vi "Configuration Editor.vi"() -> ()   [LabVIEW 2013]
doc: "This VI allows the user to create or edit an existing file located in the same directory as the the CAT Panel or the CAT Configuration Editor. It begins by opening the encrypted configuration file cat panel.cfg. The file is decrypted and then decrypted text is written to a temporary file located in the directory C:\\temp (the temporary file is called cat panel.tmp and is deleted upon successful edit of the configuration file). If the configuration file exists, then data is read into the front panel controls. When the user edits and saves the data on the front panel, the data is queued up for writing in the configuration files. Upon exit, the saved configuration data is read, the temporary file is deleted, the saved data is encrypted and written to the file cat pane.cfg."
uses:
  Type Defs/AD Settings.ctl
  Type Defs/Output Values.ctl
  Type Defs/Output Switches.ctl
  Type Defs/CO2 Settings.ctl
  Type Defs/Named Final Output name list ordered.ctl
  <vilib>/Utility/config.llb/Read Key (I32).vi
  <vilib>/Utility/config.llb/Read Key (Double).vi
  <vilib>/Utility/config.llb/Read Key (Boolean).vi
  <vilib>/Utility/config.llb/Read Key (String).vi
  <vilib>/Utility/config.llb/Write Key (I32).vi
  <vilib>/Utility/config.llb/Write Key (Double).vi
  <vilib>/Utility/config.llb/Write Key (Boolean).vi
  <vilib>/Utility/config.llb/Write Key (String).vi
  <vilib>/Utility/config.llb/NI_LVConfig.lvlib
panel:
  out "Saved?":bool
  in  "close":bool
  in  "Save":bool
  in  "tab":T1(tab)=enum."Hypoxic AD Settings"
  in  "Hyperoxic AD Settings":T2={"Set Point Force"={"A-1,  1"=inf, "A-3,  2"=inf, "A-4, 3"=inf, "A-5, 4"=5790.0, "ABCD-7, 5"=inf, "A-8, 6"=inf, "B-1,  7"=5790.0, "B-3, 8"=5790.0, "B-4,  9"=inf, "B-5, 10"=5790.0, "B-8, 11"=inf, "C-1, 12"=inf, "C-3, 13"=inf, "C-4, 14"=inf, "C-5,  15"=5790.0, "C-8, 16"=inf, "D-1, 17"=inf, "D-3, 18"=inf, "D-4,  19"=inf, "D-5,  20"=inf, "D-8,  21"=inf}, "Run A1"={"A-1,  1"=inf, "A-3,  2"=inf, "A-4, 3"=3.0, "A-5, 4"=inf, "ABCD-7, 5"=67.0, "A-8, 6"=630.0, "B-1,  7"=-30.0, "B-3, 8"=-30.0, "B-4,  9"=3.0, "B-5, 10"=inf, "B-8, 11"=630.0, "C-1, 12"=-60.0, "C-3, 13"=-60.0, "C-4, 14"=3.0, "C-5,  15"=inf, "C-8, 16"=630.0, "D-1, 17"=inf, "D-3, 18"=-30.0, "D-4,  19"=-60.0, "D-5,  20"=630.0, "D-8,  21"=930.0}, "Run A2"={"A-1,  1"=inf, "A-3,  2"=inf, "A-4, 3"=-3.0, "A-5, 4"=inf, "ABCD-7, 5"=60.0, "A-8, 6"=610.0, "B-1,  7"=-100.0, "B-3, 8"=-100.0, "B-4,  9"=-3.0, "B-5, 10"=inf, "B-8, 11"=610.0, "C-1, 12"=-120.0, "C-3, 13"=-120.0, "C-4, 14"=-3.0, "C-5,  15"=inf, "C-8, 16"=610.0, "D-1, 17"=inf, "D-3, 18"=-100.0, "D-4,  19"=-120.0, "D-5,  20"=610.0, "D-8,  21"=910.0}, "Hold A3"={"A-1,  1"=0.0, "A-3,  2"=0.0, "A-4, 3"=3.0, "A-5, 4"=inf, "ABCD-7, 5"=67.0, "A-8, 6"=630.0, "B-1,  7"=-150.0, "B-3, 8"=-150.0, "B-4,  9"=3.0, "B-5, 10"=inf, "B-8, 11"=630.0, "C-1, 12"=-300.0, "C-3, 13"=-300.0, "C-4, 14"=3.0, "C-5,  15"=inf, "C-8, 16"=630.0, "D-1, 17"=0.0, "D-3, 18"=-150.0, "D-4,  19"=-300.0, "D-5,  20"=630.0, "D-8,  21"=930.0}, "Hold A4"={"A-1,  1"=-150.0, "A-3,  2"=-150.0, "A-4, 3"=-3.0, "A-5, 4"=inf, "ABCD-7, 5"=60.0, "A-8, 6"=610.0, "B-1,  7"=-250.0, "B-3, 8"=-250.0, "B-4,  9"=-3.0, "B-5, 10"=inf, "B-8, 11"=610.0, "C-1, 12"=-500.0, "C-3, 13"=-500.0, "C-4, 14"=-3.0, "C-5,  15"=inf, "C-8, 16"=610.0, "D-1, 17"=-150.0, "D-3, 18"=-250.0, "D-4,  19"=-500.0, "D-5,  20"=610.0, "D-8,  21"=910.0}, "High AD Diff "={"A-1, 1"=FALSE, "A-3, 2"=FALSE, "A-4, 3"=FALSE, "A-5, 4"=TRUE, "ABCD-7, 5"=FALSE, "A-8, 6"=TRUE, "B-1,  7"=FALSE, "B-3, 8"=FALSE, "B-4, 9"=FALSE, "B-5, 10"=TRUE, "B-8,  11"=TRUE, "C-1, 12"=FALSE, "C-3, 13"=FALSE, "C-4,  14"=FALSE, "C-5,  15"=TRUE, "C-8, 16"=TRUE, "D-1, 17"=FALSE, "D-3, 18"=FALSE, "D-4, 19"=FALSE, "D-5,  20"=TRUE, "D-8,  21"=TRUE}, "Delay S"={"A-1,  1"=30.0, "A-3,  2"=30.0, "A-4, 3"=1.0, "A-5, 4"=1.0, "ABCD-7, 5"=1.0, "A-8, 6"=1.0, "B-1,  7"=30.0, "B-3, 8"=30.0, "B-4,  9"=1.0, "B-5, 10"=1.0, "B-8, 11"=1.0, "C-1, 12"=30.0, "C-3, 13"=30.0, "C-4, 14"=1.0, "C-5,  15"=1.0, "C-8, 16"=1.0, "D-1, 17"=30.0, "D-3, 18"=30.0, "D-4,  19"=30.0, "D-5,  20"=1.0, "D-8,  21"=1.0}}
  in  "Hyperoxic CO2 Settings":T5={"Run C1"={"A-1,  1"=inf, "A-3,  2"=inf, "A-4, 3"=9600.0, "A-5, 4"=8800.0, "ABCD-7, 5"=9800.0, "A-8, 6"=9800.0, "B-1,  7"=3400.0, "B-3, 8"=3400.0, "B-4,  9"=9600.0, "B-5, 10"=8800.0, "B-8, 11"=9800.0, "C-1, 12"=1800.0, "C-3, 13"=1800.0, "C-4, 14"=9600.0, "C-5,  15"=8800.0, "C-8, 16"=9800.0, "D-1, 17"=inf, "D-3, 18"=3400.0, "D-4,  19"=1800.0, "D-5,  20"=9800.0, "D-8,  21"=9800.0}, "Run C2"={"A-1,  1"=inf, "A-3,  2"=inf, "A-4, 3"=9500.0, "A-5, 4"=8600.0, "ABCD-7, 5"=9700.0, "A-8, 6"=9700.0, "B-1,  7"=3000.0, "B-3, 8"=3000.0, "B-4,  9"=9500.0, "B-5, 10"=8600.0, "B-8, 11"=9700.0, "C-1, 12"=1400.0, "C-3, 13"=1400.0, "C-4, 14"=9500.0, "C-5,  15"=8600.0, "C-8, 16"=9700.0, "D-1, 17"=inf, "D-3, 18"=3000.0, "D-4,  19"=1400.0, "D-5,  20"=9700.0, "D-8,  21"=9700.0}, "Hold C3"={"A-1,  1"=1800.0, "A-3,  2"=1800.0, "A-4, 3"=9000.0, "A-5, 4"=8800.0, "ABCD-7, 5"=9800.0, "A-8, 6"=9800.0, "B-1,  7"=3400.0, "B-3, 8"=3400.0, "B-4,  9"=9000.0, "B-5, 10"=8800.0, "B-8, 11"=9800.0, "C-1, 12"=1800.0, "C-3, 13"=1800.0, "C-4, 14"=9000.0, "C-5,  15"=8800.0, "C-8, 16"=9800.0, "D-1, 17"=1800.0, "D-3, 18"=3400.0, "D-4,  19"=1800.0, "D-5,  20"=9800.0, "D-8,  21"=9800.0}, "Hold C4"={"A-1,  1"=1400.0, "A-3,  2"=1400.0, "A-4, 3"=8800.0, "A-5, 4"=8600.0, "ABCD-7, 5"=9700.0, "A-8, 6"=9700.0, "B-1,  7"=3000.0, "B-3, 8"=3000.0, "B-4,  9"=8800.0, "B-5, 10"=8600.0, "B-8, 11"=9700.0, "C-1, 12"=1400.0, "C-3, 13"=1400.0, "C-4, 14"=8800.0, "C-5,  15"=8600.0, "C-8, 16"=9700.0, "D-1, 17"=1400.0, "D-3, 18"=3000.0, "D-4,  19"=1400.0, "D-5,  20"=9700.0, "D-8,  21"=9700.0}, "High CO2 Forces"={"A-1, 1"=TRUE, "A-3, 2"=TRUE, "A-4, 3"=FALSE, "A-5, 4"=TRUE, "ABCD-7, 5"=FALSE, "A-8, 6"=TRUE, "B-1,  7"=TRUE, "B-3, 8"=TRUE, "B-4, 9"=FALSE, "B-5, 10"=TRUE, "B-8,  11"=TRUE, "C-1, 12"=TRUE, "C-3, 13"=TRUE, "C-4,  14"=FALSE, "C-5,  15"=TRUE, "C-8, 16"=TRUE, "D-1, 17"=TRUE, "D-3, 18"=TRUE, "D-4, 19"=TRUE, "D-5,  20"=TRUE, "D-8,  21"=TRUE}}
  in  "AD Settings":T2={"Set Point Force"={"A-1,  1"=inf, "A-3,  2"=inf, "A-4, 3"=inf, "A-5, 4"=5790.0, "ABCD-7, 5"=inf, "A-8, 6"=inf, "B-1,  7"=5790.0, "B-3, 8"=5790.0, "B-4,  9"=inf, "B-5, 10"=5790.0, "B-8, 11"=inf, "C-1, 12"=inf, "C-3, 13"=inf, "C-4, 14"=inf, "C-5,  15"=5790.0, "C-8, 16"=inf, "D-1, 17"=inf, "D-3, 18"=inf, "D-4,  19"=inf, "D-5,  20"=inf, "D-8,  21"=inf}, "Run A1"={"A-1,  1"=inf, "A-3,  2"=inf, "A-4, 3"=3.0, "A-5, 4"=inf, "ABCD-7, 5"=67.0, "A-8, 6"=630.0, "B-1,  7"=-30.0, "B-3, 8"=-30.0, "B-4,  9"=3.0, "B-5, 10"=inf, "B-8, 11"=630.0, "C-1, 12"=-60.0, "C-3, 13"=-60.0, "C-4, 14"=3.0, "C-5,  15"=inf, "C-8, 16"=630.0, "D-1, 17"=inf, "D-3, 18"=-30.0, "D-4,  19"=-60.0, "D-5,  20"=630.0, "D-8,  21"=930.0}, "Run A2"={"A-1,  1"=inf, "A-3,  2"=inf, "A-4, 3"=-3.0, "A-5, 4"=inf, "ABCD-7, 5"=60.0, "A-8, 6"=610.0, "B-1,  7"=-100.0, "B-3, 8"=-100.0, "B-4,  9"=-3.0, "B-5, 10"=inf, "B-8, 11"=610.0, "C-1, 12"=-120.0, "C-3, 13"=-120.0, "C-4, 14"=-3.0, "C-5,  15"=inf, "C-8, 16"=610.0, "D-1, 17"=inf, "D-3, 18"=-100.0, "D-4,  19"=-120.0, "D-5,  20"=610.0, "D-8,  21"=910.0}, "Hold A3"={"A-1,  1"=0.0, "A-3,  2"=0.0, "A-4, 3"=3.0, "A-5, 4"=inf, "ABCD-7, 5"=67.0, "A-8, 6"=630.0, "B-1,  7"=-150.0, "B-3, 8"=-150.0, "B-4,  9"=3.0, "B-5, 10"=inf, "B-8, 11"=630.0, "C-1, 12"=-300.0, "C-3, 13"=-300.0, "C-4, 14"=3.0, "C-5,  15"=inf, "C-8, 16"=630.0, "D-1, 17"=0.0, "D-3, 18"=-150.0, "D-4,  19"=-300.0, "D-5,  20"=630.0, "D-8,  21"=930.0}, "Hold A4"={"A-1,  1"=-150.0, "A-3,  2"=-150.0, "A-4, 3"=-3.0, "A-5, 4"=inf, "ABCD-7, 5"=60.0, "A-8, 6"=610.0, "B-1,  7"=-250.0, "B-3, 8"=-250.0, "B-4,  9"=-3.0, "B-5, 10"=inf, "B-8, 11"=610.0, "C-1, 12"=-500.0, "C-3, 13"=-500.0, "C-4, 14"=-3.0, "C-5,  15"=inf, "C-8, 16"=610.0, "D-1, 17"=-150.0, "D-3, 18"=-250.0, "D-4,  19"=-500.0, "D-5,  20"=610.0, "D-8,  21"=910.0}, "High AD Diff "={"A-1, 1"=FALSE, "A-3, 2"=FALSE, "A-4, 3"=FALSE, "A-5, 4"=TRUE, "ABCD-7, 5"=FALSE, "A-8, 6"=TRUE, "B-1,  7"=FALSE, "B-3, 8"=FALSE, "B-4, 9"=FALSE, "B-5, 10"=TRUE, "B-8,  11"=TRUE, "C-1, 12"=FALSE, "C-3, 13"=FALSE, "C-4,  14"=FALSE, "C-5,  15"=TRUE, "C-8, 16"=TRUE, "D-1, 17"=FALSE, "D-3, 18"=FALSE, "D-4, 19"=FALSE, "D-5,  20"=TRUE, "D-8,  21"=TRUE}, "Delay S"={"A-1,  1"=30.0, "A-3,  2"=30.0, "A-4, 3"=1.0, "A-5, 4"=1.0, "ABCD-7, 5"=1.0, "A-8, 6"=1.0, "B-1,  7"=30.0, "B-3, 8"=30.0, "B-4,  9"=1.0, "B-5, 10"=1.0, "B-8, 11"=1.0, "C-1, 12"=30.0, "C-3, 13"=30.0, "C-4, 14"=1.0, "C-5,  15"=1.0, "C-8, 16"=1.0, "D-1, 17"=30.0, "D-3, 18"=30.0, "D-4,  19"=30.0, "D-5,  20"=1.0, "D-8,  21"=1.0}}
  in  "CO2 Settings":T5={"Run C1"={"A-1,  1"=inf, "A-3,  2"=inf, "A-4, 3"=9600.0, "A-5, 4"=8800.0, "ABCD-7, 5"=9800.0, "A-8, 6"=9800.0, "B-1,  7"=3400.0, "B-3, 8"=3400.0, "B-4,  9"=9600.0, "B-5, 10"=8800.0, "B-8, 11"=9800.0, "C-1, 12"=1800.0, "C-3, 13"=1800.0, "C-4, 14"=9600.0, "C-5,  15"=8800.0, "C-8, 16"=9800.0, "D-1, 17"=inf, "D-3, 18"=3400.0, "D-4,  19"=1800.0, "D-5,  20"=9800.0, "D-8,  21"=9800.0}, "Run C2"={"A-1,  1"=inf, "A-3,  2"=inf, "A-4, 3"=9500.0, "A-5, 4"=8600.0, "ABCD-7, 5"=9700.0, "A-8, 6"=9700.0, "B-1,  7"=3000.0, "B-3, 8"=3000.0, "B-4,  9"=9500.0, "B-5, 10"=8600.0, "B-8, 11"=9700.0, "C-1, 12"=1400.0, "C-3, 13"=1400.0, "C-4, 14"=9500.0, "C-5,  15"=8600.0, "C-8, 16"=9700.0, "D-1, 17"=inf, "D-3, 18"=3000.0, "D-4,  19"=1400.0, "D-5,  20"=9700.0, "D-8,  21"=9700.0}, "Hold C3"={"A-1,  1"=1800.0, "A-3,  2"=1800.0, "A-4, 3"=9000.0, "A-5, 4"=8800.0, "ABCD-7, 5"=9800.0, "A-8, 6"=9800.0, "B-1,  7"=3400.0, "B-3, 8"=3400.0, "B-4,  9"=9000.0, "B-5, 10"=8800.0, "B-8, 11"=9800.0, "C-1, 12"=1800.0, "C-3, 13"=1800.0, "C-4, 14"=9000.0, "C-5,  15"=8800.0, "C-8, 16"=9800.0, "D-1, 17"=1800.0, "D-3, 18"=3400.0, "D-4,  19"=1800.0, "D-5,  20"=9800.0, "D-8,  21"=9800.0}, "Hold C4"={"A-1,  1"=1400.0, "A-3,  2"=1400.0, "A-4, 3"=8800.0, "A-5, 4"=8600.0, "ABCD-7, 5"=9700.0, "A-8, 6"=9700.0, "B-1,  7"=3000.0, "B-3, 8"=3000.0, "B-4,  9"=8800.0, "B-5, 10"=8600.0, "B-8, 11"=9700.0, "C-1, 12"=1400.0, "C-3, 13"=1400.0, "C-4, 14"=8800.0, "C-5,  15"=8600.0, "C-8, 16"=9700.0, "D-1, 17"=1400.0, "D-3, 18"=3000.0, "D-4,  19"=1400.0, "D-5,  20"=9700.0, "D-8,  21"=9700.0}, "High CO2 Forces"={"A-1, 1"=TRUE, "A-3, 2"=TRUE, "A-4, 3"=FALSE, "A-5, 4"=TRUE, "ABCD-7, 5"=FALSE, "A-8, 6"=TRUE, "B-1,  7"=TRUE, "B-3, 8"=TRUE, "B-4, 9"=FALSE, "B-5, 10"=TRUE, "B-8,  11"=TRUE, "C-1, 12"=TRUE, "C-3, 13"=TRUE, "C-4,  14"=FALSE, "C-5,  15"=TRUE, "C-8, 16"=TRUE, "D-1, 17"=TRUE, "D-3, 18"=TRUE, "D-4, 19"=TRUE, "D-5,  20"=TRUE, "D-8,  21"=TRUE}}
  in  "Buffer":sgl=1.0 min=0 max=100
  in  "Time Offset":dbl
  out "MD5 Hash":string
  in  "Setup Menu Passwords":T6
  out "Hash 3":string
  out "Hash 2":string
  out "Hash 1":string
  in  "Lockout Date 3":timestamp format="%<%H:%M\n%x>T"
  in  "Lockout Date 2":timestamp format="%<%H:%M\n%x>T"
  in  "Lockout Date 1":timestamp format="%<%H:%M\n%x>T"
  in  "custMaxAlt":dbl caption="Customer\nMax Altitude"
  in  "Alarm Setpoints":T7={"CalLimit"=10000.0, "SenseLimit"=10000.0, "CO2Lim"=10000.0, "AltLim"=10000.0, "Low O2 "=10000.0, "High O2 offset"=10000.0}
  in  "ID":string
  in  "Setpoint":sgl=10000.0
  in  "Mode":enum8{"Off", "Stby", "Hold", "Run"}(ring)=enum."Stby"
  in  "AltCalc":bool caption="Altitude Calculation"
  in  "Channel Names":T8={"A-1, 1"="Main", "A-3, 2"="Main", "A-4, 3"="Recirculation", "A-5, 4"="Scrubber", "A-7, 5"="Oxygen", "A-8, 6"="Vent", "B-1,  7"="Boost A", "B-3, 8"="Boost A", "B-4, 9"="Recirculation", "B-5, 10"="Scrubber", "B-8, 11"="Vent", "C-1, 12"="Boost B", "C-3, 13"="Boost B", "C-4, 14"="Recirculation", "C-5,  15"="Scrubber", "C-8, 16"="Vent", "D-1, 17"="+24V", "D-3, 18"="Main", "D-4,  19"="Boost A", "D-5,  20"="Boost B", "D-8,  21"="Vent"}
  in  "AltUnits":bool caption="Altitude Units"
  in  "Max Altitude":sgl=10000.0
  in  "Other Outputs":cluster{"Alarm":bool, "Heater":bool}
  out "INI Path":path
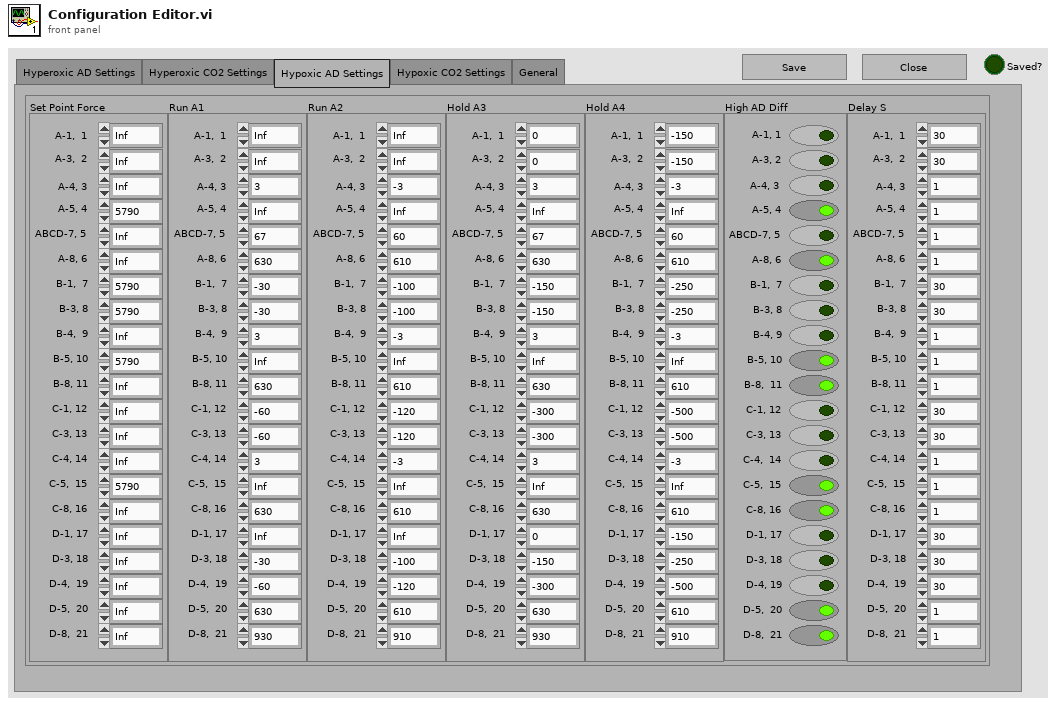
[diagram p1: front panel]
types:
  T1 = enum32{"Hyperoxic AD Settings", "Hyperoxic CO2 Settings", "Hypoxic AD Settings", "Hypoxic CO2 Settings", "General"}
  T2 = typedef "AD Settings.ctl" = cluster{"Set Point Force":T3, "Run A1":T3, "Run A2":T3, "Hold A3":T3, "Hold A4":T3, "High AD Diff ":T4, "Delay S":T3}
  T3 = typedef "Output Values.ctl" = cluster{"A-1,  1":dbl, "A-3,  2":dbl, "A-4, 3":dbl, "A-5, 4":dbl, "ABCD-7, 5":dbl, "A-8, 6":dbl, "B-1,  7":dbl, "B-3, 8":dbl, "B-4,  9":dbl, "B-5, 10":dbl, "B-8, 11":dbl, "C-1, 12":dbl, "C-3, 13":dbl, "C-4, 14":dbl, "C-5,  15":dbl, "C-8, 16":dbl, "D-1, 17":dbl, "D-3, 18":dbl, "D-4,  19":dbl, "D-5,  20":dbl, "D-8,  21":dbl}
  T4 = typedef "Output Switches.ctl" = cluster{"A-1, 1":bool, "A-3, 2":bool, "A-4, 3":bool, "A-5, 4":bool, "ABCD-7, 5":bool, "A-8, 6":bool, "B-1,  7":bool, "B-3, 8":bool, "B-4, 9":bool, "B-5, 10":bool, "B-8,  11":bool, "C-1, 12":bool, "C-3, 13":bool, "C-4,  14":bool, "C-5,  15":bool, "C-8, 16":bool, "D-1, 17":bool, "D-3, 18":bool, "D-4, 19":bool, "D-5,  20":bool, "D-8,  21":bool}
  T5 = typedef "CO2 Settings.ctl" = cluster{"Run C1":T3, "Run C2":T3, "Hold C3":T3, "Hold C4":T3, "High CO2 Forces":T4}
  T6 = cluster{"Level 1 Password":string, "Level 2 Password":string, "Level 3 Password":string}
  T7 = cluster{"CalLimit":dbl, "SenseLimit":dbl, "CO2Lim":dbl, "AltLim":dbl, "Low O2 ":dbl, "High O2 offset":dbl}
  T8 = typedef "Named Final Output name list ordered.ctl" = cluster{"A-1, 1":string, "A-3, 2":string, "A-4, 3":string, "A-5, 4":string, "A-7, 5":string, "A-8, 6":string, "B-1,  7":string, "B-3, 8":string, "B-4, 9":string, "B-5, 10":string, "B-8, 11":string, "C-1, 12":string, "C-3, 13":string, "C-4, 14":string, "C-5,  15":string, "C-8, 16":string, "D-1, 17":string, "D-3, 18":string, "D-4,  19":string, "D-5,  20":string, "D-8,  21":string}
  T9 = enum16{"open", "replace", "create", "open or create", "replace or create", "replace or create with confirmation"}
  T10 = typedef "NI_LVConfig.lvlib/Config Data RefNum.ctl" = refnum<k1>
  T11 = cluster{"Set Point Force":T3, "Run A1":T3, "Run A2":T3, "Hold A3":T3, "Hold A4":T3}
  T12 = enum16{"Left Button", "Center Button", "Right Button", "Window Close"}
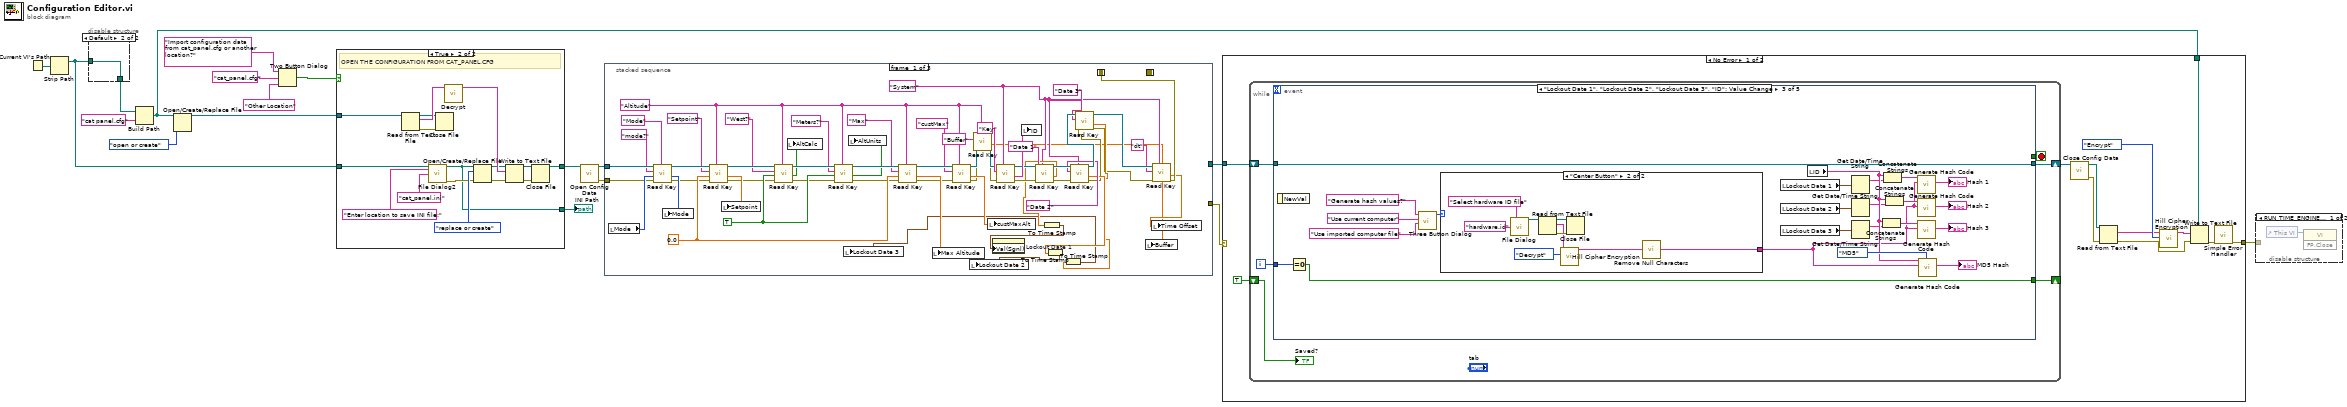
[diagram p0: block diagram]
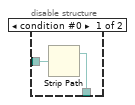
[diagram p2: hidden frame]
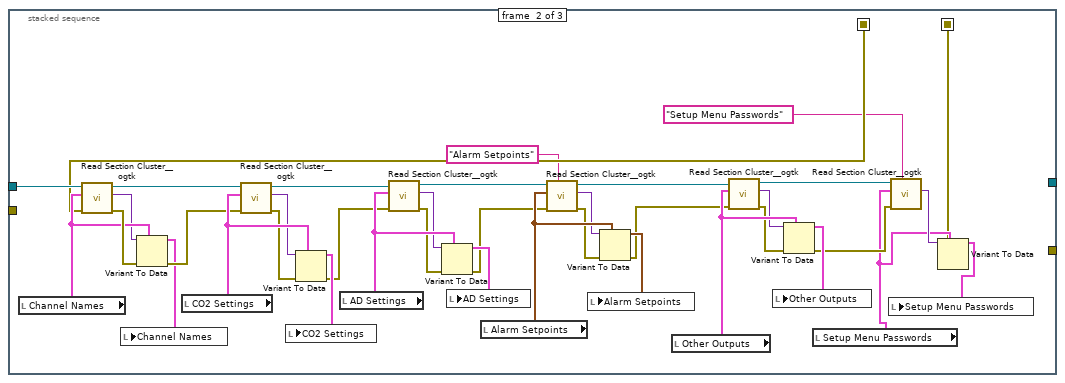
[diagram p3: hidden frame]
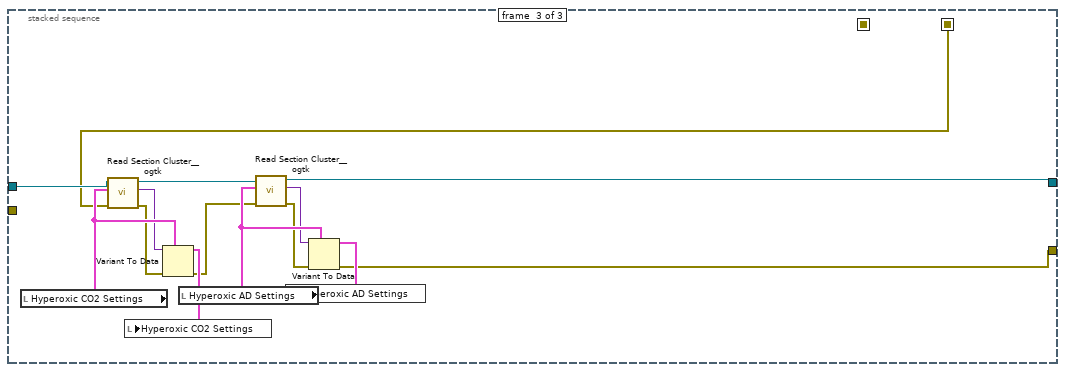
[diagram p4: hidden frame]
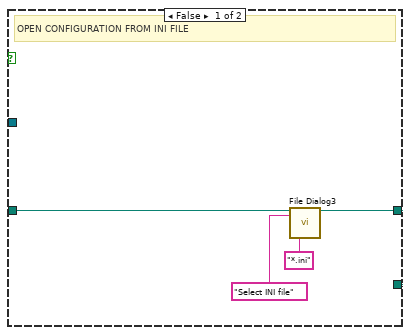
[diagram p5: hidden frame]
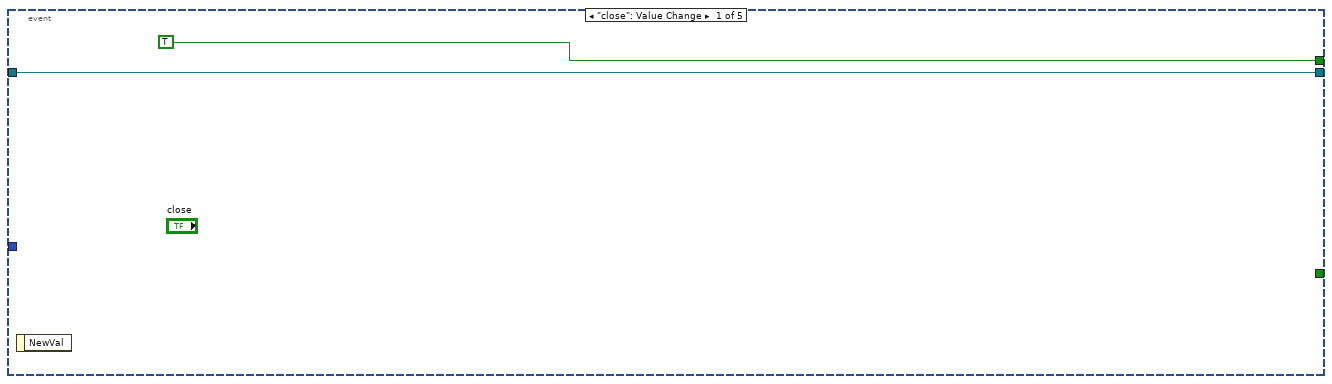
[diagram p7: hidden frame]
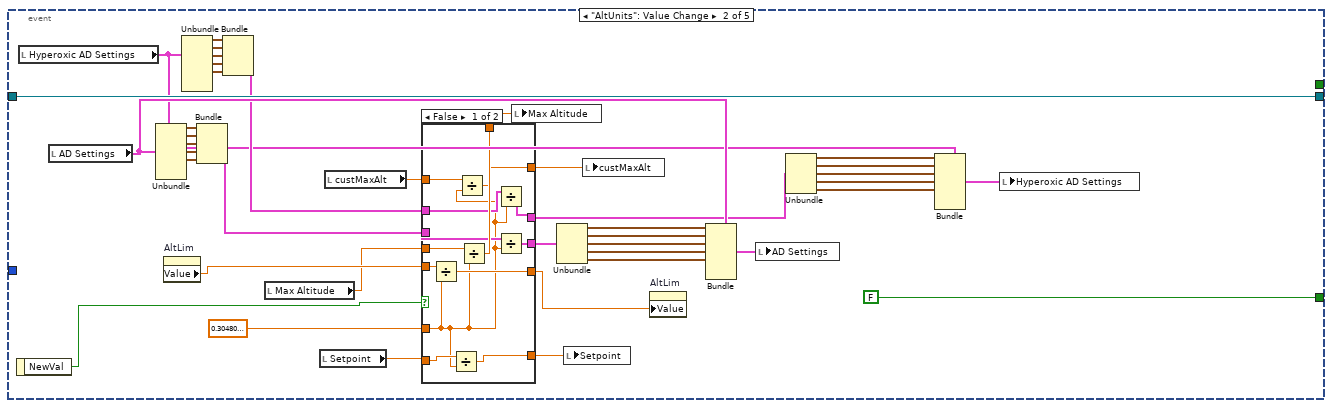
[diagram p8: hidden frame]
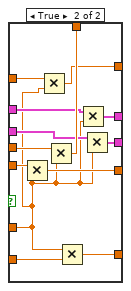
[diagram p9: hidden frame]
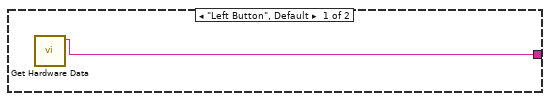
[diagram p10: hidden frame]
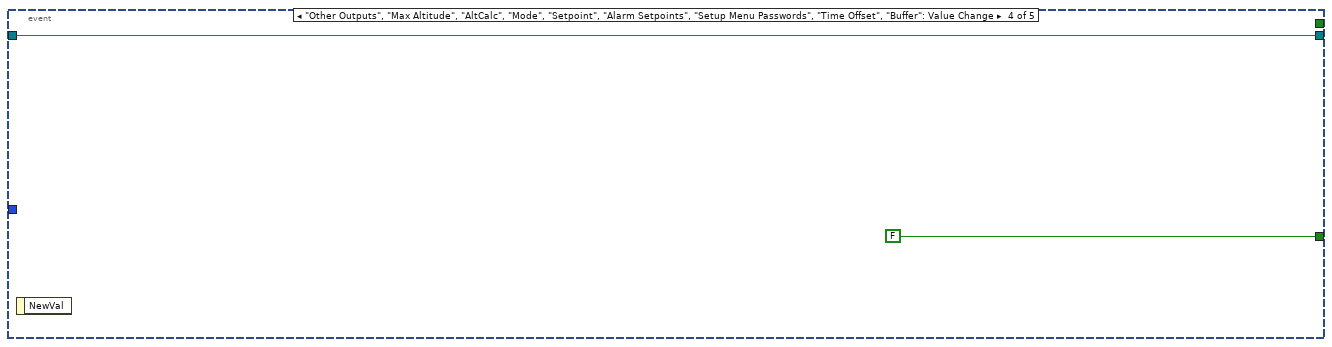
[diagram p11: hidden frame]
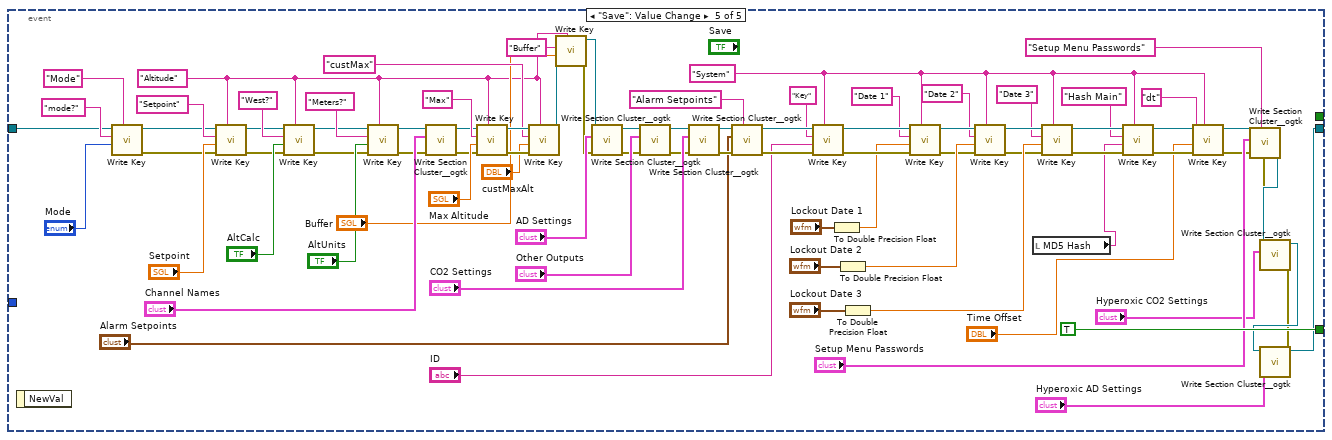
[diagram p12: hidden frame]
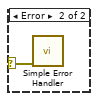
[diagram p13: hidden frame]
diagram:
  n1 = Current VI's Path() -> (path=w7:path)
  n2 = Strip Path(path=w7) -> (stripped path=w5:path)  [unwired: 1 out]
  n3 = disable-structure shown="Default" {
    disable-tunnel: w5 -> [w20 w21]
    disable-tunnel: [w19 w21] -> w8
    frame condition #0 {
      n4 = Strip Path(path=w20) -> (stripped path=w19:path)  [unwired: 1 out]
    }
    frame condition #1 (active) {
    }
  }
  n5 = Build Path(base path=w8, name or relative path="cat panel.cfg") -> (appended path=w1:path)
  n6 = Open/Create/Replace File(file path (use dialog)=w1, operation (0:open)=T9."open or create") -> (refnum out=w3:refnum<file>)  [unwired: 4 in, 2 out]
  n7 = Two Button Dialog(message="Import configuration data from cat_panel.cfg or another location?", 1:"Other Location" ("F button name (\"Cancel\")"), 2:"cat_panel.cfg" ("T button name (\"OK\")")) -> (T button?=w12:bool)
  n8 = case shown="True" w12 {
    tunnel: [w22 w26] -> w11
    tunnel: w5 -> [w23 w34]
    tunnel: w3 -> [_ w33]
    tunnel: [w22 w32] -> w4
    frame False {
      # "OPEN CONFIGURATION FROM INI FILE"
      n9 = call "File Dialog3"("start path"=w23, "prompt"="Select INI file", "pattern (all files)"="*.ini") -> ("selected path"=w22:path)  [unwired: 9 in, 3 out]
    }
    frame True {
      # "OPEN THE CONFIGURATION FROM CAT_PANEL.CFG"
      n10 = Read from Text File(file (use dialog)=w33) -> (refnum out=w31:refnum<file>, text=w38:string, error out=w30:errorcluster)  [unwired: 3 in, 1 out]
      n11 = call "File Dialog2"("start path"=w34, "prompt"="Enter location to save INI file:", "default name"="cat_panel.ini") -> ("selected path"=w32:path, "error out"=w39:errorcluster)  [unwired: 9 in, 2 out]
      n12 = Close File(refnum=w31, error in=w30) -> ()  [unwired: 2 out]
      n13 = call "Decrypt.vi"("String"=w38) -> ("Output String"=w36:string)  [unwired: 10 in]
      n14 = Open/Create/Replace File(file path (use dialog)=w32, error in=w39, operation (0:open)=T9."replace or create") -> (refnum out=w29:refnum<file>, error out=w35:errorcluster)  [unwired: 3 in, 1 out]
      n15 = Write to Text File(file (use dialog)=w29, text=w36, error in=w35) -> (refnum out=w28:refnum<file>, error out=w27:errorcluster)  [unwired: 1 in, 1 out]
      n16 = Close File(refnum=w28, error in=w27) -> (path=w26:path)  [unwired: 1 out]
    }
  }
  "INI Path" <- w4
  n17 = call <vilib>:"Open Config Data.vi"("configuration file path"=w11) -> ("error out"=w9:errorcluster, "refnum"=w10:T10)  [unwired: 8 in, 1 out]
  n18 = stacked-sequence {
    seq-local: [w50 _ _] -> [_ w108 _]
    seq-local: [_ w100 _] -> [_ _ w138]
    tunnel: w10 -> [w99 w117 w141]
    tunnel: w9 -> [w80 _ _]
    tunnel: [_ _ w140] -> w18
    tunnel: [_ _ w139] -> w17
    frame #0 {
      w54 = "System" ("section")
      w85 = sgl 0.0
      w86 = TRUE
      w44 = "Altitude" ("section")
      n19 = local read "Mode"() -> (w94:enum8{"Off", "Stby", "Hold", "Run"})
      n20 = call-poly <vilib>:"Read Key.vi"("section"="Mode", "error in (no error)"=w80, "default value"=w94, "key"="mode?", "refnum"=w99) -> ("error out"=w79:errorcluster, "value"=w93:i32, "refnum out"=w98:T10)  [unwired: 3 in, 1 out]
      n21 = local write "Mode"(w93) -> ()
      n22 = call-poly <vilib>:"Read Key.vi"("section"=w44, "error in (no error)"=w79, "default value"=w85, "key"="Setpoint", "refnum"=w98) -> ("error out"=w78:errorcluster, "value"=w84:dbl, "refnum out"=w97:T10)  [unwired: 3 in, 1 out]
      n23 = local write "Setpoint"(w84) -> ()
      n24 = call-poly <vilib>:"Read Key.vi"("section"=w44, "error in (no error)"=w78, "default value"=w86, "key"="West?", "refnum"=w97) -> ("error out"=w77:errorcluster, "value"=w81:bool, "refnum out"=w96:T10)  [unwired: 3 in, 1 out]
      n25 = local write "AltCalc"(w81) -> ()
      n26 = call-poly <vilib>:"Read Key.vi"("section"=w44, "error in (no error)"=w77, "default value"=w86, "key"="Meters?", "refnum"=w96) -> ("error out"=w76:errorcluster, "value"=w82:bool, "refnum out"=w95:T10)  [unwired: 3 in, 1 out]
      n27 = local write "AltUnits"(w82) -> ()
      n28 = call-poly <vilib>:"Read Key.vi"("section"=w44, "error in (no error)"=w76, "default value"=w85, "key"="Max", "refnum"=w95) -> ("error out"=w72:errorcluster, "value"=w83:dbl, "refnum out"=w73:T10)  [unwired: 3 in, 1 out]
      n29 = local write "Max Altitude"(w83) -> ()
      n30 = call-poly <vilib>:"Read Key.vi"("section"=w44, "error in (no error)"=w72, "key"="custMax", "refnum"=w73) -> ("error out"=w46:errorcluster, "value"=w70:dbl, "refnum out"=w48:T10)  [unwired: 4 in, 1 out]
      n31 = call-poly <vilib>:"Read Key.vi"("section"=w44, "error in (no error)"=w46, "key"="Buffer", "refnum"=w48) -> ("error out"=w45:errorcluster, "value"=w42:dbl, "refnum out"=w47:T10)  [unwired: 4 in, 1 out]
      n32 = local write "custMaxAlt"(w70) -> ()
      n33 = call-poly <vilib>:"Read Key.vi"("section"=w54, "error in (no error)"=w45, "key"="Key", "refnum"=w47) -> ("error out"=w66:errorcluster, "value"=w74:string, "refnum out"=w69:T10)  [unwired: 4 in, 1 out]
      n34 = local write "ID"(w74) -> ()
      n35 = call-poly <vilib>:"Read Key.vi"("section"=w54, "error in (no error)"=w66, "key"="Date 1", "refnum"=w69) -> ("error out"=w65:errorcluster, "value"=w61:dbl, "refnum out"=w68:T10)  [unwired: 4 in, 1 out]
      n36 = To Time Stamp(1:w61) -> (0:w56:timestamp)
      n37 = property on="Lockout Date 1" class="AbsTime (strict)"("Val(Sgnl)"=w56) -> ()  [unwired: 2 in, 2 out]
      n38 = call-poly <vilib>:"Read Key.vi"("section"=w54, "error in (no error)"=w65, "key"="Date 2", "refnum"=w68) -> ("error out"=w52:errorcluster, "value"=w60:dbl, "refnum out"=w67:T10)  [unwired: 4 in, 1 out]
      n39 = To Time Stamp(1:w60) -> (0:w59:timestamp)
      n40 = local write "Lockout Date 2"(w59) -> ()
      n41 = call-poly <vilib>:"Read Key.vi"("section"=w54, "error in (no error)"=w52, "key"="Date 3", "refnum"=w67) -> ("error out"=w51:errorcluster, "value"=w58:dbl, "refnum out"=w55:T10)  [unwired: 4 in, 1 out]
      n42 = To Time Stamp(1:w58) -> (0:w57:timestamp)
      n43 = local write "Lockout Date 3"(w57) -> ()
      n44 = local write "Buffer"(w42) -> ()
      n45 = call-poly <vilib>:"Read Key.vi"("section"=w54, "error in (no error)"=w51, "key"="dt", "refnum"=w55) -> ("error out"=w50:errorcluster, "value"=w49:dbl)  [unwired: 4 in, 2 out]
      n46 = local write "Time Offset"(w49) -> ()
    }
    frame #1 {
      n47 = local read "Channel Names"() -> (w123:T8)
      n48 = call <userlib>:"Read Section Cluster__ogtk.vi"("error in (no error)"=w108, "Section Formatted Cluster Type"=w123, "refnum"=w117) -> ("error out"=w125:errorcluster, "Section Formatted Cluster"=w122:variant, "dup refnum"=w118:T10)  [unwired: 4 in, 2 out]
      n49 = Variant To Data(error in=w125, type=w123, Variant=w122) -> (data=w124:T8, error out=w126:errorcluster)
      n50 = local write "Channel Names"(w124) -> ()
      n51 = local read "CO2 Settings"() -> (w128:T5)
      n52 = call <userlib>:"Read Section Cluster__ogtk.vi"("error in (no error)"=w126, "Section Formatted Cluster Type"=w128, "refnum"=w118) -> ("error out"=w115:errorcluster, "Section Formatted Cluster"=w127:variant, "dup refnum"=w119:T10)  [unwired: 4 in, 2 out]
      n53 = Variant To Data(error in=w115, type=w128, Variant=w127) -> (data=w129:T5, error out=w114:errorcluster)
      n54 = local write "CO2 Settings"(w129) -> ()
      n55 = local read "AD Settings"() -> (w131:T2)
      n56 = call <userlib>:"Read Section Cluster__ogtk.vi"("error in (no error)"=w114, "Section Formatted Cluster Type"=w131, "refnum"=w119) -> ("error out"=w113:errorcluster, "Section Formatted Cluster"=w130:variant, "dup refnum"=w120:T10)  [unwired: 4 in, 2 out]
      n57 = Variant To Data(error in=w113, type=w131, Variant=w130) -> (data=w132:T2, error out=w112:errorcluster)
      n58 = local write "AD Settings"(w132) -> ()
      n59 = local read "Alarm Setpoints"() -> (w134:T7)
      n60 = call <userlib>:"Read Section Cluster__ogtk.vi"("section (optional)"="Alarm Setpoints", "error in (no error)"=w112, "Section Formatted Cluster Type"=w134, "refnum"=w120) -> ("error out"=w111:errorcluster, "Section Formatted Cluster"=w133:variant, "dup refnum"=w121:T10)  [unwired: 3 in, 2 out]
      n61 = Variant To Data(error in=w111, type=w134, Variant=w133) -> (data=w135:T7, error out=w110:errorcluster)
      n62 = local write "Alarm Setpoints"(w135) -> ()
      n63 = local read "Other Outputs"() -> (w137:cluster{"Alarm":bool, "Heater":bool})
      n64 = call <userlib>:"Read Section Cluster__ogtk.vi"("error in (no error)"=w110, "Section Formatted Cluster Type"=w137, "refnum"=w121) -> ("error out"=w109:errorcluster, "Section Formatted Cluster"=w136:variant, "dup refnum"=w105:T10)  [unwired: 4 in, 2 out]
      n65 = Variant To Data(error in=w109, type=w137, Variant=w136) -> (data=w116:cluster{"Alarm":bool, "Heater":bool}, error out=w106:errorcluster)
      n66 = local write "Other Outputs"(w116) -> ()
      n67 = local read "Setup Menu Passwords"() -> (w102:T6)
      n68 = call <userlib>:"Read Section Cluster__ogtk.vi"("section (optional)"="Setup Menu Passwords", "error in (no error)"=w106, "Section Formatted Cluster Type"=w102, "refnum"=w105) -> ("Section Formatted Cluster"=w103:variant)  [unwired: 3 in, 4 out]
      n69 = Variant To Data(type=w102, Variant=w103) -> (data=w101:T6, error out=w100:errorcluster)  [unwired: 1 in]
      n70 = local write "Setup Menu Passwords"(w101) -> ()
    }
    frame #2 {
      n71 = local read "Hyperoxic CO2 Settings"() -> (w147:T5)
      n72 = call <userlib>:"Read Section Cluster__ogtk.vi"("error in (no error)"=w138, "Section Formatted Cluster Type"=w147, "refnum"=w141) -> ("error out"=w144:errorcluster, "Section Formatted Cluster"=w146:variant, "dup refnum"=w145:T10)  [unwired: 4 in, 2 out]
      n73 = Variant To Data(error in=w144, type=w147, Variant=w146) -> (data=w148:T5, error out=w143:errorcluster)
      n74 = local write "Hyperoxic CO2 Settings"(w148) -> ()
      n75 = local read "Hyperoxic AD Settings"() -> (w150:T2)
      n76 = call <userlib>:"Read Section Cluster__ogtk.vi"("error in (no error)"=w143, "Section Formatted Cluster Type"=w150, "refnum"=w145) -> ("error out"=w142:errorcluster, "Section Formatted Cluster"=w149:variant, "dup refnum"=w140:T10)  [unwired: 4 in, 2 out]
      n77 = Variant To Data(error in=w142, type=w150, Variant=w149) -> (data=w151:T2, error out=w139:errorcluster)
      n78 = local write "Hyperoxic AD Settings"(w151) -> ()
    }
  }
  n79 = case shown="No Error" w17 {
    selector: w17 -> [_ w358]
    tunnel: w18 -> [w161 _]
    tunnel: w1 -> [w154 _]
    tunnel: [w152 _] -> w16
    frame No Error {
      n80 = while {
        shift-right: [w167] -> w162
        shift-left: w161 -> [w168]
        shift-right: [w166] -> _
        shift-left: TRUE -> [w165]
        i -> [w164]
        stop <- w169 stop-if-true
        n81 = event shown="[2] \"Lockout Date 1\", \"Lockout Date 2\", \"Lockout Date 3\", \"ID\": Value Change" {
          selector: _ -> [_ _ _ _ _]
          dyn-events: _ -> [_ _ _ _ _]
          timeout: _ -> [_ _ _ _ _]
          tunnel: [TRUE _ _ _ _] -> w169
          tunnel: w168 -> [w170 w211 w256 w272 w343]
          tunnel: [w170 w211 w256 w272 w282] -> w167
          tunnel: [_ FALSE w254 FALSE TRUE] -> w166
          tunnel: w164 -> [_ _ w255 _ _]
          event "close": Value Change {
            n82 = event-data() -> ()  [unwired: 1 in, 1 out]
          }
          event "AltUnits": Value Change {
            n83 = event-data() -> ("NewVal"=w203:bool)  [unwired: 1 in]
            n84 = local read "Hyperoxic AD Settings"() -> (w172:T2)
            n85 = local read "AD Settings"() -> (w193:T2)
            n86 = Unbundle(w193) -> ("Set Point Force"=w199:T3, "Run A1"=w198:T3, "Run A2"=w197:T3, "Hold A3"=w196:T3, "Hold A4"=w195:T3)  [unwired: 2 out]
            n87 = property on="AltLim" class="DigNum (strict)"() -> ("Value"=w209:dbl)  [unwired: 2 in, 2 out]
            n88 = Unbundle(w172) -> ("Set Point Force"=w182:T3, "Run A1"=w183:T3, "Run A2"=w184:T3, "Hold A3"=w185:T3, "Hold A4"=w181:T3)  [unwired: 2 out]
            n89 = Bundle("Set Point Force"=w199, "Run A1"=w198, "Run A2"=w197, "Hold A3"=w196, "Hold A4"=w195) -> (w194:T11)  [unwired: 1 in]
            n90 = Bundle("Set Point Force"=w182, "Run A1"=w183, "Run A2"=w184, "Hold A3"=w185, "Hold A4"=w181) -> (w180:T11)  [unwired: 1 in]
            n91 = local read "Max Altitude"() -> (w205:sgl)
            n92 = local read "Setpoint"() -> (w206:sgl)
            n93 = local read "custMaxAlt"() -> (w201:dbl)
            n94 = case shown="False" w203 {
              tunnel: w209 -> [w223 w236]
              tunnel: [w224 w237] -> w208
              tunnel: sgl 0.3048 ("y") -> [w213 w226]
              tunnel: w205 -> [w222 w235]
              tunnel: [w221 w234] -> w204
              tunnel: w194 -> [w220 w233]
              tunnel: [w219 w232] -> w191
              tunnel: w206 -> [w218 w231]
              tunnel: [w217 w230] -> w207
              tunnel: w201 -> [w216 w229]
              tunnel: [w215 w228] -> w200
              tunnel: w180 -> [w214 w227]
              tunnel: [w212 w225] -> w173
              frame False {
                n95 = Divide(x=w223, y=w213) -> (x/y=w224:dbl)
                n96 = Divide(x=w218, y=w213) -> (x/y=w217:sgl)
                n97 = Divide(x=w216, y=w213) -> (x/y=w215:dbl)
                n98 = Divide(x=w222, y=w213) -> (x/y=w221:sgl)
                n99 = Divide(x=w214, y=w213) -> (x/y=w212:T11)
                n100 = Divide(x=w220, y=w213) -> (x/y=w219:T11)
              }
              frame True {
                n101 = Multiply(x=w236, y=w226) -> (x*y=w237:dbl)
                n102 = Multiply(x=w229, y=w226) -> (x*y=w228:dbl)
                n103 = Multiply(x=w235, y=w226) -> (x*y=w234:sgl)
                n104 = Multiply(x=w226, y=w231) -> (x*y=w230:sgl)
                n105 = Multiply(x=w227, y=w226) -> (x*y=w225:T11)
                n106 = Multiply(x=w233, y=w226) -> (x*y=w232:T11)
              }
            }
            n107 = local write "Max Altitude"(w204) -> ()
            n108 = Unbundle(w191) -> ("Set Point Force"=w190:T3, "Run A1"=w189:T3, "Run A2"=w188:T3, "Hold A3"=w187:T3, "Hold A4"=w186:T3)
            n109 = local write "Setpoint"(w207) -> ()
            n110 = local write "custMaxAlt"(w200) -> ()
            n111 = property on="AltLim" class="DigNum (strict)"("Value"=w208) -> ()  [unwired: 2 in, 2 out]
            n112 = Bundle(cluster=w193, "Set Point Force"=w190, "Run A1"=w189, "Run A2"=w188, "Hold A3"=w187, "Hold A4"=w186) -> (w192:T2)  [unwired: 2 in]
            n113 = local write "AD Settings"(w192) -> ()
            n114 = Unbundle(w173) -> ("Set Point Force"=w175:T3, "Run A1"=w176:T3, "Run A2"=w177:T3, "Hold A3"=w178:T3, "Hold A4"=w179:T3)
            n115 = Bundle(cluster=w172, "Set Point Force"=w175, "Run A1"=w176, "Run A2"=w177, "Hold A3"=w178, "Hold A4"=w179) -> (w174:T2)  [unwired: 2 in]
            n116 = local write "Hyperoxic AD Settings"(w174) -> ()
          }
          event "Lockout Date 1", "Lockout Date 2", "Lockout Date 3", "ID": Value Change {
            n117 = event-data() -> ()  [unwired: 1 in, 1 out]
            n118 = Equal To 0?(x=w255) -> (x = 0?=w254:bool)
            n119 = call <vilib>:"Three Button Dialog.vi"("Center Button Text (\"No\")"="Use imported computer file" ("Center Button Text (\"No\")"), "Left Button Text (\"Yes\")"="Use current computer" ("Left Button Text (\"Yes\")"), "message"="Generate hash values?") -> ("Which Button?"=w257:T12)  [unwired: 8 in]
            n120 = case shown="\"Center Button\"" w257 {
              tunnel: [w261 w262] -> w238
              frame "Left Button", Default {
                n121 = call "Get Hardware Data.vi"() -> ("Fingerprint"=w261:string)  [unwired: 11 in]
              }
              frame "Center Button" {
                n122 = call "File Dialog"("prompt"="Select hardware ID file", "default name"="hardware.id") -> ("selected path"=w267:path)  [unwired: 10 in, 3 out]
                n123 = Read from Text File(file (use dialog)=w267) -> (refnum out=w265:refnum<file>, text=w264:string, error out=w266:errorcluster)  [unwired: 3 in, 1 out]
                n124 = call <userlib>:"Hill Cipher Encryption.vi"("Operation"=enum16{"Encrypt", "Decrypt", "Decrypt from Hex"}."Decrypt", "Input String"=w264) -> ("Output String"=w263:string)  [unwired: 7 in, 2 out]
                n125 = Close File(refnum=w265, error in=w266) -> ()  [unwired: 2 out]
                n126 = call "Remove Null Characters.vi"("strIn"=w263) -> ("strOut"=w262:string)  [unwired: 4 in]
              }
            }
            n127 = local read "Lockout Date 1"() -> (w239:timestamp)
            n128 = local read "Lockout Date 2"() -> (w240:timestamp)
            n129 = local read "Lockout Date 3"() -> (w241:timestamp)
            n130 = local read "ID"() -> (w251:string)
            n131 = Get Date/Time String(seconds (now)=w239) -> (date string=w242:string)  [unwired: 2 in, 1 out]
            n132 = Get Date/Time String(seconds (now)=w240) -> (date string=w243:string)  [unwired: 2 in, 1 out]
            n133 = Get Date/Time String(seconds (now)=w241) -> (date string=w244:string)  [unwired: 2 in, 1 out]
            n134 = Concatenate Strings(w251, w244) -> (w247:string)
            n135 = Concatenate Strings(w251, w242) -> (w245:string)
            n136 = Concatenate Strings(w251, w243) -> (w246:string)
            n137 = call "Generate Hash Code.vi"("Fingerprint"=w238, "Product ID"=w245) -> ("Hash"=→"Hash 1":string)  [unwired: 8 in, 1 out]
            n138 = call "Generate Hash Code.vi"("Fingerprint"=w238, "Product ID"=w246) -> ("Hash"=→"Hash 2":string)  [unwired: 8 in, 1 out]
            n139 = call "Generate Hash Code.vi"("Fingerprint"=w238, "Product ID"=w247) -> ("Hash"=→"Hash 3":string)  [unwired: 8 in, 1 out]
            n140 = call "Generate Hash Code.vi"("Hash"=enum16{"MD5", "FNV-1"}."MD5", "Fingerprint"=w238, "Product ID"=w251) -> ("Hash"=→"MD5 Hash":string)  [unwired: 7 in, 1 out]
          }
          event "Other Outputs", "Max Altitude", "AltCalc", "Mode", "Setpoint", "Alarm Setpoints", "Setup Menu Passwords", "Time Offset", "Buffer": Value Change {
            n141 = event-data() -> ()  [unwired: 1 in, 1 out]
          }
          event "Save": Value Change {
            w289 = "System" ("section")
            w275 = "Altitude" ("section")
            n142 = event-data() -> ()  [unwired: 1 in, 1 out]
            n143 = call-poly <vilib>:"Write Key.vi"("section"="Mode", "value"="Mode", "key"="mode?", "refnum"=w343) -> ("error out"=w325:errorcluster, "refnum out"=w345:T10)  [unwired: 5 in, 1 out]
            n144 = call-poly <vilib>:"Write Key.vi"("section"=w275, "error in (no error)"=w325, "value"="Setpoint", "key"="Setpoint", "refnum"=w345) -> ("error out"=w326:errorcluster, "refnum out"=w347:T10)  [unwired: 4 in, 1 out]
            n145 = call-poly <vilib>:"Write Key.vi"("section"=w275, "error in (no error)"=w326, "value"="AltCalc", "key"="West?", "refnum"=w347) -> ("error out"=w327:errorcluster, "refnum out"=w350:T10)  [unwired: 4 in, 1 out]
            n146 = call-poly <vilib>:"Write Key.vi"("section"=w275, "error in (no error)"=w327, "value"="AltUnits", "key"="Meters?", "refnum"=w350) -> ("error out"=w328:errorcluster, "refnum out"=w351:T10)  [unwired: 4 in, 1 out]
            n147 = call <userlib>:"Write Section Cluster__ogtk.vi"("error in (no error)"=w328, "Section Formatted Cluster"="Channel Names", "refnum"=w351) -> ("error out"=w329:errorcluster, "dup refnum"=w353:T10)  [unwired: 7 in]
            n148 = call-poly <vilib>:"Write Key.vi"("section"=w275, "error in (no error)"=w329, "value"="Max Altitude", "key"="Max", "refnum"=w353) -> ("error out"=w315:errorcluster, "refnum out"=w316:T10)  [unwired: 4 in, 1 out]
            n149 = call-poly <vilib>:"Write Key.vi"("section"=w275, "error in (no error)"=w315, "value"="custMaxAlt", "key"="custMax", "refnum"=w316) -> ("error out"=w280:errorcluster, "refnum out"=w281:T10)  [unwired: 4 in, 1 out]
            n150 = call-poly <vilib>:"Write Key.vi"("section"=w275, "error in (no error)"=w280, "value"="Buffer", "key"="Buffer", "refnum"=w281) -> ("error out"=w278:errorcluster, "refnum out"=w279:T10)  [unwired: 4 in, 1 out]
            n151 = call <userlib>:"Write Section Cluster__ogtk.vi"("error in (no error)"=w278, "Section Formatted Cluster"="AD Settings", "refnum"=w279) -> ("error out"=w330:errorcluster, "dup refnum"=w356:T10)  [unwired: 7 in]
            n152 = call <userlib>:"Write Section Cluster__ogtk.vi"("error in (no error)"=w330, "Section Formatted Cluster"="Other Outputs", "refnum"=w356) -> ("error out"=w331:errorcluster, "dup refnum"=w355:T10)  [unwired: 7 in]
            n153 = call <userlib>:"Write Section Cluster__ogtk.vi"("error in (no error)"=w331, "Section Formatted Cluster"="CO2 Settings", "refnum"=w355) -> ("error out"=w332:errorcluster, "dup refnum"=w333:T10)  [unwired: 7 in]
            n154 = call <userlib>:"Write Section Cluster__ogtk.vi"("section (optional)"="Alarm Setpoints", "error in (no error)"=w332, "Section Formatted Cluster"="Alarm Setpoints", "refnum"=w333) -> ("error out"=w323:errorcluster, "dup refnum"=w324:T10)  [unwired: 6 in]
            n155 = call-poly <vilib>:"Write Key.vi"("section"=w289, "error in (no error)"=w323, "value"="ID", "key"="Key", "refnum"=w324) -> ("error out"=w317:errorcluster, "refnum out"=w318:T10)  [unwired: 4 in, 1 out]
            n156 = To Double Precision Float(number="Lockout Date 1") -> (double precision float=w306:dbl)
            n157 = To Double Precision Float(number="Lockout Date 2") -> (double precision float=w304:dbl)
            n158 = To Double Precision Float(number="Lockout Date 3") -> (double precision float=w302:dbl)
            n159 = call-poly <vilib>:"Write Key.vi"("section"=w289, "error in (no error)"=w317, "value"=w306, "key"="Date 1", "refnum"=w318) -> ("error out"=w300:errorcluster, "refnum out"=w311:T10)  [unwired: 4 in, 1 out]
            n160 = call-poly <vilib>:"Write Key.vi"("section"=w289, "error in (no error)"=w300, "value"=w304, "key"="Date 2", "refnum"=w311) -> ("error out"=w301:errorcluster, "refnum out"=w310:T10)  [unwired: 4 in, 1 out]
            n161 = local read "MD5 Hash"() -> (w294:string)
            n162 = call-poly <vilib>:"Write Key.vi"("section"=w289, "error in (no error)"=w301, "value"=w302, "key"="Date 3", "refnum"=w310) -> ("error out"=w296:errorcluster, "refnum out"=w297:T10)  [unwired: 4 in, 1 out]
            n163 = call-poly <vilib>:"Write Key.vi"("section"=w289, "error in (no error)"=w296, "value"=w294, "key"="Hash Main", "refnum"=w297) -> ("error out"=w290:errorcluster, "refnum out"=w291:T10)  [unwired: 4 in, 1 out]
            n164 = call-poly <vilib>:"Write Key.vi"("section"=w289, "error in (no error)"=w290, "value"="Time Offset", "key"="dt", "refnum"=w291) -> ("error out"=w293:errorcluster, "refnum out"=w292:T10)  [unwired: 4 in, 1 out]
            n165 = call <userlib>:"Write Section Cluster__ogtk.vi"("section (optional)"="Setup Menu Passwords", "error in (no error)"=w293, "Section Formatted Cluster"="Setup Menu Passwords", "refnum"=w292) -> ("error out"=w274:errorcluster, "dup refnum"=w286:T10)  [unwired: 6 in]
            n166 = call <userlib>:"Write Section Cluster__ogtk.vi"("error in (no error)"=w274, "Section Formatted Cluster"="Hyperoxic CO2 Settings", "refnum"=w286) -> ("error out"=w273:errorcluster, "dup refnum"=w284:T10)  [unwired: 7 in]
            n167 = call <userlib>:"Write Section Cluster__ogtk.vi"("error in (no error)"=w273, "Section Formatted Cluster"="Hyperoxic AD Settings", "refnum"=w284) -> ("dup refnum"=w282:T10)  [unwired: 7 in, 1 out]
          }
        }
        "Saved?" <- w165
      }
      n168 = call <vilib>:"Close Config Data.vi"("refnum"=w162) -> ("error out"=w159:errorcluster, "file path"=w160:path)  [unwired: 9 in]
      n169 = Read from Text File(file (use dialog)=w160, error in=w159) -> (text=w156:string, error out=w158:errorcluster)  [unwired: 2 in, 2 out]
      n170 = call <userlib>:"Hill Cipher Encryption.vi"("Operation"=enum16{"Encrypt", "Decrypt", "Decrypt from Hex"}."Encrypt", "Input String"=w156) -> ("Output String"=w155:string)  [unwired: 7 in, 2 out]
      n171 = Write to Text File(file (use dialog)=w154, text=w155, error in=w158) -> (error out=w153:errorcluster)  [unwired: 1 in, 2 out]
      n172 = call <vilib>:"Simple Error Handler.vi"("error in (no error)"=w153) -> ("error out"=w152:errorcluster)  [unwired: 4 in, 4 out]
    }
    frame Error {
      n173 = call <vilib>:"Simple Error Handler.vi"("error in (no error)"=w358) -> ()  [unwired: 4 in, 5 out]
    }
  }
  n174 = disable-structure shown="RUN_TIME_ENGINE==True" {
    disable-tunnel: w16 -> [_ _]
    frame condition #0 {
      n175 = control-ref of="This VI"() -> (w359:refnum<vi>)
      n176 = invoke class="VI" method="FP.Close"(reference=w359) -> ()  [unwired: 2 in, 3 out]
    }
    frame condition #1 (active) {
    }
  }
